vi "Test WS Server.vi"() -> ()   [LabVIEW 2020]
uses:
  Stream-Websocket/Websocket Server/Websocket Server.lvclass
  C:/Program Files (x86)/National Instruments/LabVIEW 2020/vi.lib/IlluminatedG/lv-stream/Endpoint/Endpoint.lvclass
  <vilib>/IlluminatedG/lv-stream/stream/Stream.lvclass/Stream.ctl
  <vilib>/IlluminatedG/lv-stream/stream/Dispatch Sniffer Data.vi
  <vilib>/IlluminatedG/lv-stream/stream/Prepared.vi
  <vilib>/IlluminatedG/lv-stream/Endpoint/Cast Sniffer Callback.vi
  <vilib>/Utility/error.llb/Error Cluster From Error Code.vi
  Stream-Websocket/Websocket Client/Websocket Client.lvclass
  <vilib>/IlluminatedG/lv-stream/stream/Stream.lvclass
  <vilib>/IlluminatedG/IG HTTP Utils/HTTP Utils/Request/Request.lvclass
  <vilib>/IlluminatedG/IG HTTP Utils/HTTP Utils/Response/Response.lvclass
  <vilib>/IlluminatedG/lv-stream/Endpoint/Endpoint.lvclass
panel:
  in  "HTTP Port":u16=7080
  out "WS":errorcluster
  out "HTTP":errorcluster
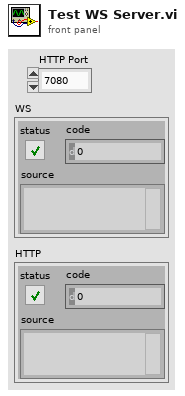
[diagram p1: front panel]
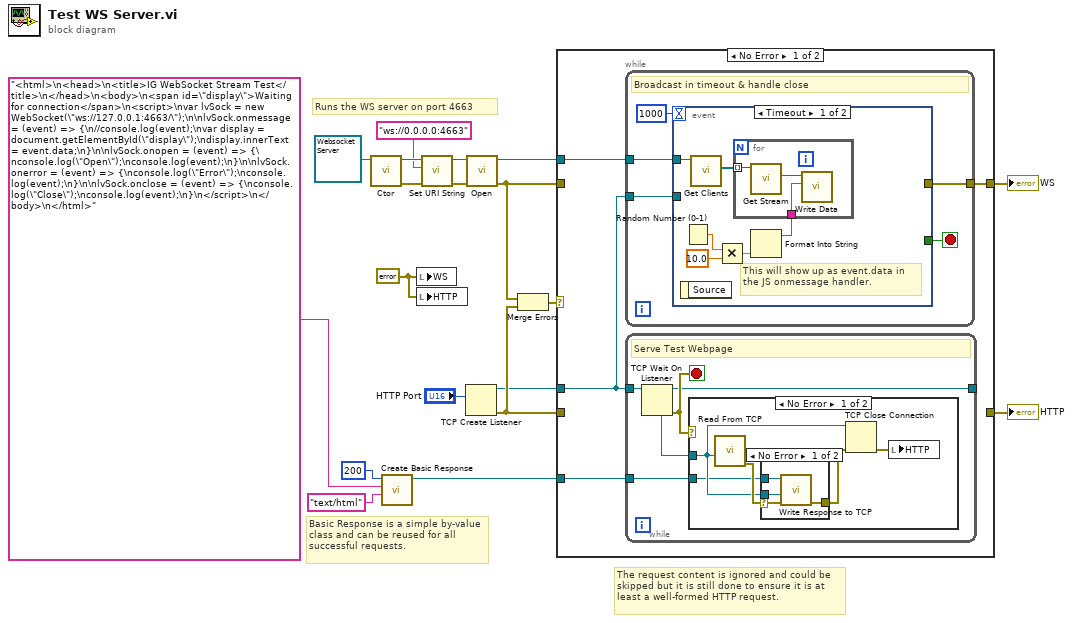
[diagram p0: block diagram]
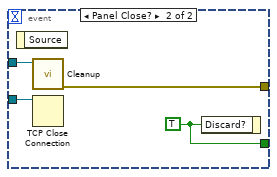
[diagram p2: hidden frame]
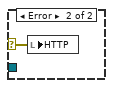
[diagram p4: hidden frame]
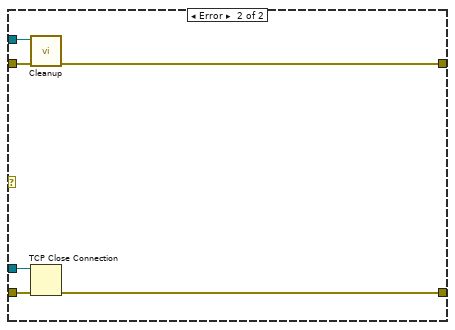
[diagram p5: hidden frame]
diagram:
  w7 = errorcluster {"status"=FALSE, "code"=0, "source"=""} ("WS")
  # "The request content is ignored and could be skipped but it is still done to ensure it is at least a well-formed HTTP request."
  # "Basic Response is a simple by-value class and can be reused for all successful requests."
  # "Runs the WS server on port 4663"
  n1 = call-dynamic "Ctor.vi"("Websocket Server in"=refnum<class "Websocket Server.lvclass"> refnum) -> ("error out"=w11:errorcluster, "Websocket Server out"=w13:refnum<class "Websocket Server.lvclass">)  [unwired: 9 in]
  n2 = call <vilib>:"Create Basic Response.vi"("Content-Type (text/plain)"="text/html", "Payload"="<html>\n<head>\n<title>IG WebSocket Stream Test</title>\n</head>\n<body>\n<span id=\"display\">Waiting for connection</span>\n<script>\nvar lvSock = new WebSocket(\"ws://127.0.0.1:4663/\");\n\nlvSock.onmessage = (event) => {\n//console.log(event);\nvar display = document.getElementById(\"display\");\ndisplay.innerText = event.data;\n}\n\nlvSock.onopen = (event) => {\nconsole.log(\"Open\");\nconsole.log(event);\n}\n\nlvSock.onerror = (event) => {\nconsole.log(\"Error\");\nconsole.log(event);\n}\n\nlvSock.onclose = (event) => {\nconsole.log(\"Close\");\nconsole.log(event);\n}\n</script>\n</body>\n</html>", "Status Code"=u16 200) -> ("Response out"=w16:refnum<class "Response.lvclass">)  [unwired: 7 in, 1 out]
  n3 = local write "WS"(w7) -> ()
  n4 = local write "HTTP"(w7) -> ()
  n5 = call <vilib>:"Set URI String.vi"("error in (no error)"=w11, "URI String"="ws://0.0.0.0:4663", "Endpoint in"=w13) -> ("error out"=w8:errorcluster, "Endpoint out"=w9:refnum<class "Websocket Server.lvclass">)  [unwired: 7 in]
  n6 = TCP Create Listener(10:"HTTP Port") -> (0:w19:errorcluster, 3:w5:refnum<k5>)  [unwired: 4 in, 1 out]
  n7 = call <vilib>:"Open.vi"("error in (no error)"=w8, "Endpoint in"=w9) -> ("error out"=w4:errorcluster, "Endpoint out"=w10:refnum<class "Websocket Server.lvclass">)  [unwired: 8 in]
  n8 = Merge Errors(w4, w19) -> (w3:errorcluster)
  n9 = case shown="No Error" w3 {
    tunnel: w16 -> [w23 _]
    tunnel: w10 -> [w22 w62]
    tunnel: w5 -> [w21 w60]
    tunnel: w4 -> [_ w63]
    tunnel: w19 -> [_ w59]
    tunnel: [_ w58] -> w2
    tunnel: [w20 w61] -> w1
    frame No Error {
      n10 = while {
        tunnel: w21 -> [w28]
        tunnel: w22 -> [w26]
        tunnel: [w24] -> w20
        stop <- w27 stop-if-true
        # "Broadcast in timeout & handle close"
        n11 = event shown="[0] Timeout" {
          selector: _ -> [_ _]
          dyn-events: _ -> [_ _]
          timeout: 1000 -> [_ _]
          tunnel: w28 -> [_ w41]
          tunnel: [_ w40] -> w27
          tunnel: w26 -> [w34 w39]
          tunnel: [_ w38] -> w24
          event Timeout {
            # "This will show up as event.data in the JS onmessage handler."
            n12 = event-data() -> ()  [unwired: 1 in, 1 out]
            n13 = Random Number (0-1)() -> (number: 0 to 1=w33:dbl)
            n14 = call "Get Clients.vi"("Websocket Server in"=w34) -> ("Clients"=w30:refnum<class "Websocket Client.lvclass">[])  [unwired: 8 in, 2 out]
            n15 = Multiply(x=w33, y=10.0) -> (x*y=w31:dbl)
            n16 = Format Into String(w31) -> (resulting string=w29:string)  [unwired: 3 in, 1 out]
            n17 = for {
              tunnel: w30 -> [w36] mode=indexing
              tunnel: w29 -> [w37]
              n18 = call-dynamic "Get Stream.vi"("Websocket Client in"=w36) -> ("Stream"=w35:refnum<class "Stream.lvclass">)  [unwired: 8 in, 2 out]
              n19 = call <vilib>:"Write Data.vi"("Data"=w37, "Stream in"=w35) -> ()  [unwired: 8 in, 2 out]
            }
          }
          event Panel Close? {
            w40 = TRUE ("Discard?")
            n20 = event-data() -> ()  [unwired: 1 in, 1 out]
            n21 = call-dynamic "Cleanup.vi"("Websocket Server in"=w39) -> ("error out"=w38:errorcluster)  [unwired: 10 in]
            n22 = TCP Close Connection(connection ID=w41) -> ()  [unwired: 2 in, 2 out]
            n23 = event-data("Discard?"=w40) -> ()  [unwired: 1 in, 1 out]
          }
        }
      }
      n24 = while {
        tunnel: w21 -> [w46]
        tunnel: w23 -> [w43]
        tunnel: [w42] -> _
        stop <- w45 stop-if-true
        # "Serve Test Webpage"
        n25 = TCP Wait On Listener(11:w46) -> (0:w45:errorcluster, 3:w42:refnum<k5>, 4:w44:refnum<k5>)  [unwired: 3 in, 2 out]
        n26 = case shown="No Error" w45 {
          selector: w45 -> [_ w57]
          tunnel: w44 -> [w50 _]
          tunnel: w43 -> [w48 _]
          frame No Error {
            n27 = call <vilib>:"Read From TCP.vi"("TCP Connection"=w50) -> ("error out"=w51:errorcluster)  [unwired: 9 in, 1 out]
            n28 = case shown="No Error" w51 {
              selector: w51 -> [w55 w56]
              tunnel: w48 -> [w54 _]
              tunnel: w50 -> [w53 _]
              tunnel: [w52 w56] -> w49
              frame No Error {
                n29 = call <vilib>:"Write Response to TCP.vi"("error in (no error)"=w55, "TCP Connection"=w53, "Response in"=w54) -> ("error out"=w52:errorcluster)  [unwired: 7 in, 1 out]
              }
              frame Error {
              }
            }
            n30 = TCP Close Connection(connection ID=w50, error in (no error)=w49) -> (error out=w47:errorcluster)  [unwired: 1 in, 1 out]
            n31 = local write "HTTP"(w47) -> ()
          }
          frame Error {
            n32 = local write "HTTP"(w57) -> ()
          }
        }
      }
    }
    frame Error {
      n33 = call-dynamic "Cleanup.vi"("error in (no error)"=w63, "Websocket Server in"=w62) -> ("error out"=w61:errorcluster)  [unwired: 9 in]
      n34 = TCP Close Connection(connection ID=w60, error in (no error)=w59) -> (error out=w58:errorcluster)  [unwired: 1 in, 1 out]
    }
  }
  "WS" <- w1
  "HTTP" <- w2
